vi "Delete Uint32Array DVR.vi"(8 "error in (no error)":errorcluster, 11 "Uint32Array DVR in":refnum<data-value>) -> (0 "error out":errorcluster, 3 "Uint32Array out":refnum<class "Uint32Array.lvclass">)   [LabVIEW 2015, in "MDSplus.lvlib" / "Uint32Array.lvclass"]
uses:
  <vilib>/MDSplus/Classes/Data_Class/Array_Class/Uint32Array_Class/Uint32Array.lvclass
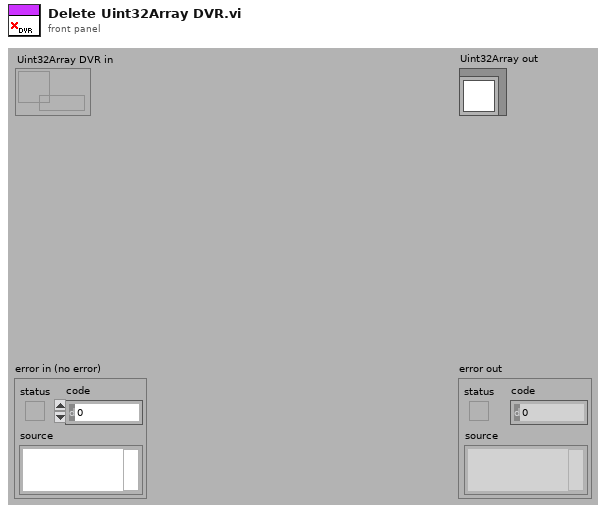
[diagram p1: front panel]
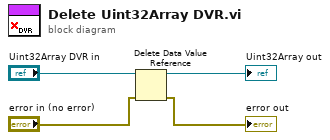
[diagram p0: block diagram]
diagram:
  n1 = Delete Data Value Reference(data value reference="Uint32Array DVR in", error in="error in (no error)") -> (data value=→"Uint32Array out":refnum<class "Uint32Array.lvclass">, error out=→"error out":errorcluster)
